vi "test_play_wav.vi"() -> ()   [LabVIEW 2019]
panel:
  in  "wait":u32=4 caption="sec"
  out "path":path
  out "status":bool
  in  "problem":enum16{"OK", "Warning", "Error"}(ring)=enum."Error"
  out "error out":errorcluster
  # "The wait is necessary because \"play_wav.vi\" does not wait for the sound finished."
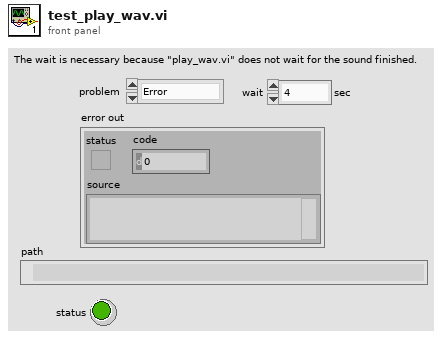
[diagram p1: front panel]
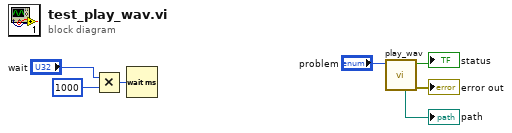
[diagram p0: block diagram]
diagram:
  n1 = Multiply(x="wait", y=u32 1000) -> (x*y=w3:u32)
  n2 = Wait (ms)(milliseconds to wait=w3) -> ()  [unwired: 1 out]
  n3 = call "play_wav.vi"("problem"="problem") -> ("error out"=→"error out":errorcluster, "status"=→"status":bool, "path"=→"path":path)  [unwired: 8 in]
